vi "BT Example 3 - Sequence with Failure.vi"() -> ()   [LabVIEW 2021]
uses:
  Support/Nodes/abs_Node/Status.ctl
  Blackboard/Blackboard.lvclass
  Support/Nodes/Decorators/Repeater/Support/Finish On - Type.ctl
  System/bt_System.lvclass
  Blackboard/Blackboard.lvclass/Blackboard.ctl
  Support/Nodes/Leaves/abs_Type Leaf/abs_Type Leaf.lvclass/abs_Type Leaf.ctl
  Blackboard/Get Value Type/Get I32.vi
  Blackboard/Get Value Type/Get Boolean.vi
  <vilib>/TSA/Abstract Data Classes/Abs_Types/I32 Integer/Static Read.vi
  <vilib>/TSA/Abstract Data Classes/Abs_Types/Boolean/Static Read.vi
  Blackboard/Support/Index Group.vi
  Blackboard/Support/Index Tags.vi
  Support/Nodes/Leaves/abs_Type Leaf/Properties/Write Value Class.vi
  <vilib>/TSA/Abstract Data Classes/Abs_Types/Boolean/Abs_Boolean.lvclass
  C:/Program Files (x86)/National Instruments/LabVIEW 2021/vi.lib/TSA/Abstract Data Classes/Abs_Types/Value/Abs_Value.lvclass
  C:/Program Files (x86)/National Instruments/LabVIEW 2021/vi.lib/TSA/Abstract Data Classes/Abs_Types/Type/Abs_Type.lvclass
  <vilib>/TSA/Omni-Bus/Local Bus/Support/Bool/Local Bus_Boolean.lvclass
  <vilib>/TSA/Omni-Bus/Local Bus/Support/I32/Local Bus_I32.lvclass
  <vilib>/TSA/Abstract Data Classes/Abs_Types/I32 Integer/Abs_I32 Integer.lvclass
  Support/Nodes/Leaves/Test Boolean/Test Abs_Boolean.lvclass
  C:/Users/Tim/Documents/GitHub/LV_Behaviour_Tree/Source/Support/Nodes/abs_Node/bt_Node.lvclass
  C:/Users/Tim/Documents/GitHub/LV_Behaviour_Tree/Source/Support/Nodes/Leaves/abs_Type Leaf/abs_Type Leaf.lvclass
  <vilib>/TSA/Omni-Bus/Local Bus/Support/Initialise DVR's.vi
  <vilib>/TSA/Abstract Data Classes/Constants/Support/Bool/Bool.vi
  <vilib>/TSA/Abstract Data Classes/Functions/Math/Support/Increment/I32/Method.vi
  <vilib>/TSA/Abstract Data Classes/Functions/Compare/Support/Less/I32/Method_Const.vi
  <vilib>/TSA/Abstract Data Classes/Abs_Types/Value/Abs_Value.lvclass
  <vilib>/TSA/Abstract Data Classes/Abs_Types/Type/Abs_Type.lvclass
  <vilib>/TSA/Omni-Bus/Local Bus/Support/DBL/Local Bus_DBL.lvclass
  <vilib>/TSA/Omni-Bus/Local Bus/Support/SGL/Local Bus_SGL.lvclass
  <vilib>/TSA/Omni-Bus/Local Bus/Support/EXT/Local Bus_EXT.lvclass
  <vilib>/TSA/Omni-Bus/Local Bus/Support/STR/Local Bus_String.lvclass
  <vilib>/TSA/Omni-Bus/Local Bus/Support/Variant/Local Bus_Variant.lvclass
  <vilib>/TSA/Omni-Bus/Local Bus/Support/WFM/Local Bus_Waveform.lvclass
  <vilib>/TSA/Omni-Bus/Local Bus/Support/Time/Local Bus_Time.lvclass
  <vilib>/TSA/Omni-Bus/Local Bus/Support/U8/Local Bus_U8.lvclass
  <vilib>/TSA/Omni-Bus/Local Bus/Support/U16/Local Bus_U16.lvclass
  <vilib>/TSA/Omni-Bus/Local Bus/Support/U32/Local Bus_U32.lvclass
  <vilib>/TSA/Omni-Bus/Local Bus/Support/U64/Local Bus_U64.lvclass
  <vilib>/TSA/Omni-Bus/Local Bus/Support/I8/Local Bus_I8.lvclass
  <vilib>/TSA/Omni-Bus/Local Bus/Support/I16/Local Bus_I16.lvclass
  <vilib>/TSA/Omni-Bus/Local Bus/Support/I64/Local Bus_I64.lvclass
  <vilib>/TSA/Omni-Bus/Local Bus/Support/CSGL/Local Bus_CSGL.lvclass
  <vilib>/TSA/Omni-Bus/Local Bus/Support/CDBL/Local Bus_CDBL.lvclass
  <vilib>/TSA/Omni-Bus/Local Bus/Support/CEXT/Local Bus_CEXT.lvclass
  BT.lvlib
  Support/Nodes/Decorators/Repeater/bt_Repeater.lvclass
  <vilib>/TSA/Abstract Data Classes/Constants/Support/Bool/Const_Bool.lvclass
  Support/Nodes/abs_Node/bt_Node.lvclass
  <vilib>/TSA/Abstract Data Classes/Functions/Math/Support/Increment/I32/Increment_I32.lvclass
  <vilib>/TSA/Abstract Data Classes/Functions/Compare/Support/Less/I32/Less_I32.lvclass
panel:
  out "Count":i32
  out "Status":T1
  out "Indicators":bool[](array[boolean])
  in  "stop":bool
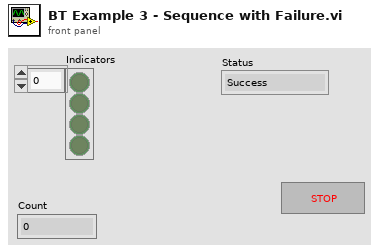
[diagram p1: front panel]
types:
  T1 = typedef "BT.lvlib/bt_Node.lvclass/Status.ctl" = enum16{"Success", "Failure", "Running"}
  T2 = typedef "BT.lvlib/bt_Repeater.lvclass/Finish On - Type.ctl" = enum16{"Success", "Failure", "Never"}
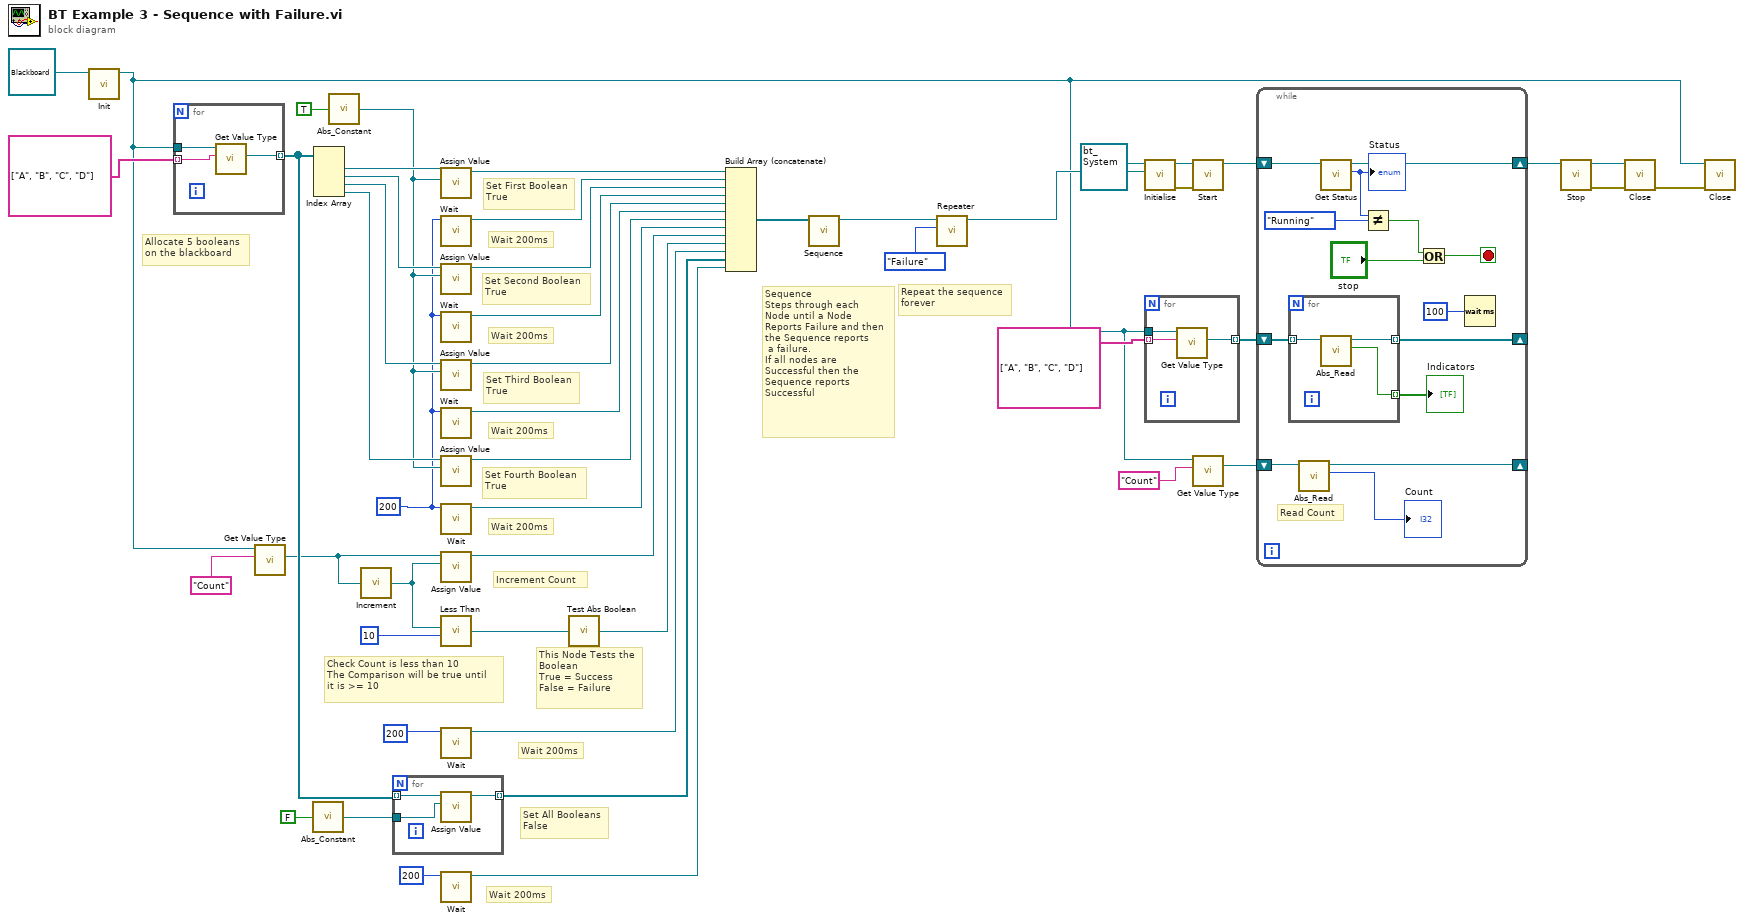
[diagram p0: block diagram]
diagram:
  w13 = u32 200 ("Time (ms)")
  # "Wait 200ms"
  # "This Node Tests the\nBoolean\nTrue = Success\nFalse = Failure"
  # "Check Count is less than 10\nThe Comparison will be true until\nit is >= 10"
  # "Increment Count"
  # "Wait 200ms"
  # "Wait 200ms"
  # "Wait 200ms"
  # "Wait 200ms"
  # "Wait 200ms"
  # "Set All Booleans\nFalse"
  # "Set Fourth Boolean\nTrue"
  # "Set Third Boolean\nTrue"
  # "Set Second Boolean\nTrue"
  # "Set First Boolean\nTrue"
  # "Allocate 5 booleans\non the blackboard"
  # "Repeat the sequence\nforever"
  # "Sequence\nSteps through each\nNode until a Node\nReports Failure and then\nthe Sequence reports\n a failure.\nIf all nodes are \nSuccessful then the \nSequence reports \nSuccessful"
  n1 = call-dynamic "Init.vi"("bt_Blackboard in"=refnum<class "Blackboard.lvclass"> refnum) -> ("bt_Blackboard out"=w3:refnum<class "Blackboard.lvclass">)  [unwired: 9 in, 1 out]
  n2 = for {
    tunnel: w3 -> [w52]
    tunnel: string[] ["A", "B", "C", "D"] ("Tag") -> [w51] mode=indexing
    tunnel: [w50] -> w17 mode=indexing
    n3 = call-poly "Get Value Type.vi"("Tag"=w51, "Blackboard in"=w52) -> ("Value"=w50:refnum<class "Abs_Boolean.lvclass">)  [unwired: 6 in, 3 out]
  }
  n4 = call-poly "Get Value Type.vi"("Tag"="Count", "Blackboard in"=w3) -> ("Value"=w8:refnum<class "Abs_I32 Integer.lvclass">)  [unwired: 6 in, 3 out]
  n5 = call-poly <vilib>:"Abs_Constant.vi"("Boolean"=FALSE) -> ("Abs_Boolean.lvclass"=w19:refnum<class "Abs_Boolean.lvclass">)  [unwired: 4 in]
  n6 = Index Array(array=w17) -> (element #1=w32:refnum<class "Abs_Boolean.lvclass">, element #2=w29:refnum<class "Abs_Boolean.lvclass">, element #3=w26:refnum<class "Abs_Boolean.lvclass">, element #4=w24:refnum<class "Abs_Boolean.lvclass">)  [unwired: 4 in]
  n7 = call-poly <vilib>:"Abs_Constant.vi"("Boolean"=TRUE) -> ("Abs_Boolean.lvclass"=w23:refnum<class "Abs_Boolean.lvclass">)  [unwired: 4 in]
  n8 = call-poly <vilib>:"Increment.vi"("Value"=w8) -> ("Result"=w7:refnum<class "Abs_I32 Integer.lvclass">)  [unwired: 4 in]
  n9 = for {
    tunnel: w19 -> [w55]
    tunnel: w17 -> [w54] mode=indexing
    tunnel: [w53] -> w16 mode=indexing
    n10 = call "Assign Value.vi"("Assigned Value"=w55, "Value"=w54) -> ("Node Out"=w53:refnum<class "bt_Node.lvclass">)  [unwired: 9 in]
  }
  n11 = call "Assign Value.vi"("Assigned Value"=w23, "Value"=w32) -> ("Node Out"=w33:refnum<class "bt_Node.lvclass">)  [unwired: 9 in]
  n12 = call "Wait.vi"("Time (ms)"=w13) -> ("Node Out"=w30:refnum<class "bt_Node.lvclass">)  [unwired: 10 in]
  n13 = call "Assign Value.vi"("Assigned Value"=w23, "Value"=w29) -> ("Node Out"=w28:refnum<class "bt_Node.lvclass">)  [unwired: 9 in]
  n14 = call "Wait.vi"("Time (ms)"=w13) -> ("Node Out"=w27:refnum<class "bt_Node.lvclass">)  [unwired: 10 in]
  n15 = call "Assign Value.vi"("Assigned Value"=w23, "Value"=w26) -> ("Node Out"=w25:refnum<class "bt_Node.lvclass">)  [unwired: 9 in]
  n16 = call "Wait.vi"("Time (ms)"=w13) -> ("Node Out"=w22:refnum<class "bt_Node.lvclass">)  [unwired: 10 in]
  n17 = call "Assign Value.vi"("Assigned Value"=w23, "Value"=w24) -> ("Node Out"=w21:refnum<class "bt_Node.lvclass">)  [unwired: 9 in]
  n18 = call "Wait.vi"("Time (ms)"=w13) -> ("Node Out"=w20:refnum<class "bt_Node.lvclass">)  [unwired: 10 in]
  n19 = call "Assign Value.vi"("Assigned Value"=w7, "Value"=w8) -> ("Node Out"=w11:refnum<class "bt_Node.lvclass">)  [unwired: 9 in]
  n20 = call-poly <vilib>:"Less Than.vi"("Value"=10, "Value A"=w7) -> ("Result"=w10:refnum<class "Abs_Boolean.lvclass">)  [unwired: 4 in]
  n21 = call "Wait.vi"("Time (ms)"=u32 200) -> ("Node Out"=w1:refnum<class "bt_Node.lvclass">)  [unwired: 10 in]
  n22 = call "Wait.vi"("Time (ms)"=u32 200) -> ("Node Out"=w15:refnum<class "bt_Node.lvclass">)  [unwired: 10 in]
  n23 = call "Test Abs Boolean.vi"("Abs_Boolean.lvclass"=w10) -> ("abs_Node"=w9:refnum<class "bt_Node.lvclass">)  [unwired: 4 in]
  n24 = Build Array (concatenate)(w33, w30, w28, w27, w25, w22, w21, w20, w11, w9, w1, w16, w15) -> (w35:refnum<class "bt_Node.lvclass">[])
  n25 = call "Sequence.vi"("Nodes"=w35) -> ("Node"=w36:refnum<class "bt_Node.lvclass">)  [unwired: 10 in]
  n26 = call "Repeater.vi"("Finish On"=Finish_On_-_Type."Failure", "Node In"=w36) -> ("Node Out"=w38:refnum<class "bt_Node.lvclass">)  [unwired: 9 in]
  n27 = call "Initialise.vi"("Behaviour Tree"=w38, "bt_System in"=refnum<class "bt_System.lvclass"> refnum) -> ("error out"=w39:errorcluster, "bt_System out"=w40:refnum<class "bt_System.lvclass">)  [unwired: 8 in]
  n28 = for {
    tunnel: string[] ["A", "B", "C", "D"] ("Tag") -> [w58] mode=indexing
    tunnel: [w57] -> w44 mode=indexing
    tunnel: w3 -> [w56]
    n29 = call-poly "Get Value Type.vi"("Tag"=w58, "Blackboard in"=w56) -> ("Value"=w57:refnum<class "Abs_Boolean.lvclass">)  [unwired: 6 in, 3 out]
  }
  n30 = call "Start.vi"("error in (no error)"=w39, "bt_System in"=w40) -> ("bt_System out"=w49:refnum<class "bt_System.lvclass">)  [unwired: 8 in, 1 out]
  n31 = call-poly "Get Value Type.vi"("Tag"="Count", "Blackboard in"=w3) -> ("Value"=w5:refnum<class "Abs_I32 Integer.lvclass">)  [unwired: 6 in, 3 out]
  n32 = while {
    shift-right: [w67] -> w48
    shift-left: w49 -> [w68]
    shift-right: [w71] -> _
    shift-left: w44 -> [w72]
    shift-right: [w59] -> _
    shift-left: w5 -> [w60]
    stop <- w65 stop-if-true
    # "Read Count"
    n33 = for {
      tunnel: w72 -> [w75] mode=indexing
      tunnel: [w74] -> w71 mode=indexing
      tunnel: [w73] -> w70 mode=indexing
      n34 = call-poly <vilib>:"Abs_Read.vi"("Abs_Boolean in"=w75) -> ("Boolean"=w73:bool, "Abs_Boolean out"=w74:refnum<class "Abs_Boolean.lvclass">)  [unwired: 8 in, 1 out]
    }
    "Indicators" <- w70
    n35 = call-poly <vilib>:"Abs_Read.vi"("Abs_I32 Integer in"=w60) -> ("Value"=→"Count":i32, "Abs_I32 Integer out"=w59:refnum<class "Abs_I32 Integer.lvclass">)  [unwired: 8 in, 1 out]
    n36 = call "Get Status.vi"("bt_System in"=w68) -> ("Status"=w64:T1, "bt_System out"=w67:refnum<class "bt_System.lvclass">)  [unwired: 8 in, 1 out]
    "Status" <- w64
    n37 = Not Equal?(x=w64, y=Status."Running") -> (x != y?=w62:bool)
    n38 = Or(x=w62, y="stop") -> (x .or. y?=w65:bool)
    n39 = Wait (ms)(milliseconds to wait=u32 100) -> ()  [unwired: 1 out]
  }
  n40 = call "Stop.vi"("bt_System in"=w48) -> ("error out"=w41:errorcluster, "bt_System out"=w42:refnum<class "bt_System.lvclass">)  [unwired: 9 in]
  n41 = call-dynamic "Close.vi"("error in (no error)"=w41, "bt_System in"=w42) -> ("error out"=w47:errorcluster)  [unwired: 8 in, 1 out]
  n42 = call-dynamic "Close.vi"("error in (no error)"=w47, "bt_Blackboard in"=w3) -> ()  [unwired: 8 in, 2 out]
